vi "Read Mapping buffer.vi"(8 "error in (no error)":errorcluster, 11 "Buffers in":refnum<class "CV-Buffers.lvclass">) -> (0 "error out":errorcluster, 2 "Mapping buffer":refnum<queue>, 3 "Buffers out":refnum<class "CV-Buffers.lvclass">)   [LabVIEW 2013, in "CameraVision.lvlib" / "CV-Buffers.lvclass"]
uses:
  CV-Buffers.lvclass
  Mapping-buffer.ctl
  Temperature/Temperature-characteristics.ctl
  Analysis/Characteristics-cluster.ctl
  CV-Buffers.lvclass/CV-Buffers.ctl
  Temperature/CV-Temperature.lvclass
  Analysis/CV-Analysis.lvclass
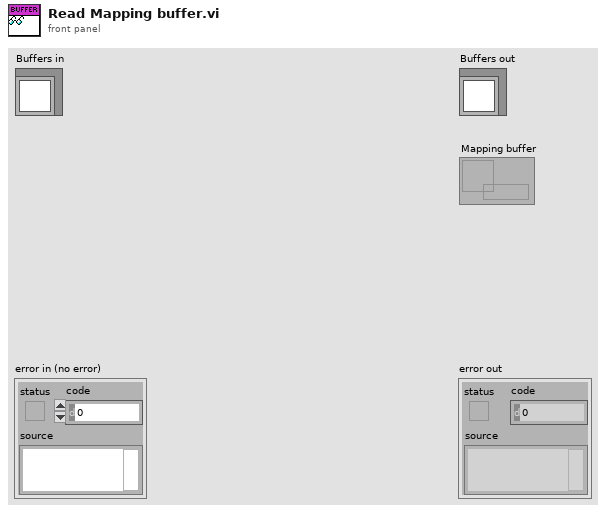
[diagram p1: front panel]
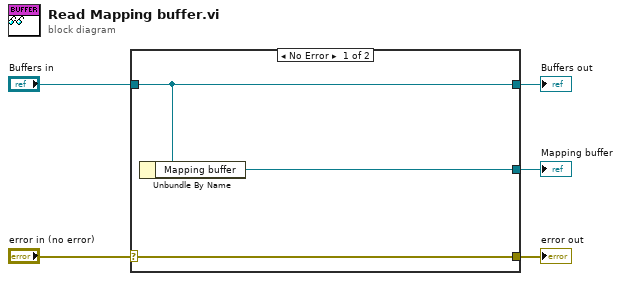
[diagram p0: block diagram]
diagram:
  n1 = case shown="No Error" "error in (no error)" {
    selector: "error in (no error)" -> [w8 w9]
    tunnel: [w8 w9] -> w4
    tunnel: [w7 w10] -> w2
    tunnel: "Buffers in" -> [w7 w10]
    tunnel: [w6 _] -> w1
    frame No Error {
      n2 = Unbundle By Name(w7) -> ("Mapping buffer"=w6:refnum<queue>)
    }
    frame Error {
    }
  }
  "error out" <- w4
  "Buffers out" <- w2
  "Mapping buffer" <- w1
